vi "Process Messages.vi"(8 "error in (no error)":errorcluster, 11 "Effect in":refnum<class "Effect.lvclass">) -> (0 "error out":errorcluster, 3 "Effect out":refnum<class "Effect.lvclass">)   [LabVIEW 2018, in "Effect.lvclass"]
uses:
  Effect.lvclass
  Effect.lvclass/Effect.ctl
  20a259b6-a1a0-4479-baf0-259017fe30d7.vi
  bbb3d459-c080-460f-b42f-ee43debab906.vi
  Libraries/Messaging/Messaging.lvlib
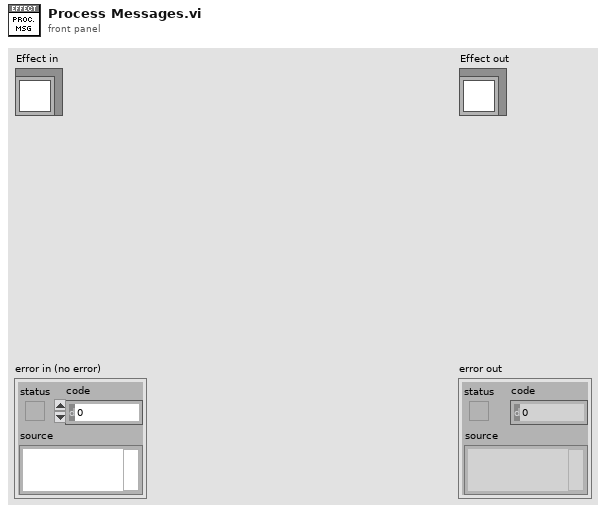
[diagram p1: front panel]
types:
  T1 = typedef "Messaging.lvlib/Message Cluster.ctl" = cluster{"Event":string, "Source":string, "Target":string, "Data":variant}
  T2 = typedef "Audio Processing.lvlib/Value Properties.ctl" = cluster{"Lower":dbl, "Upper":dbl}
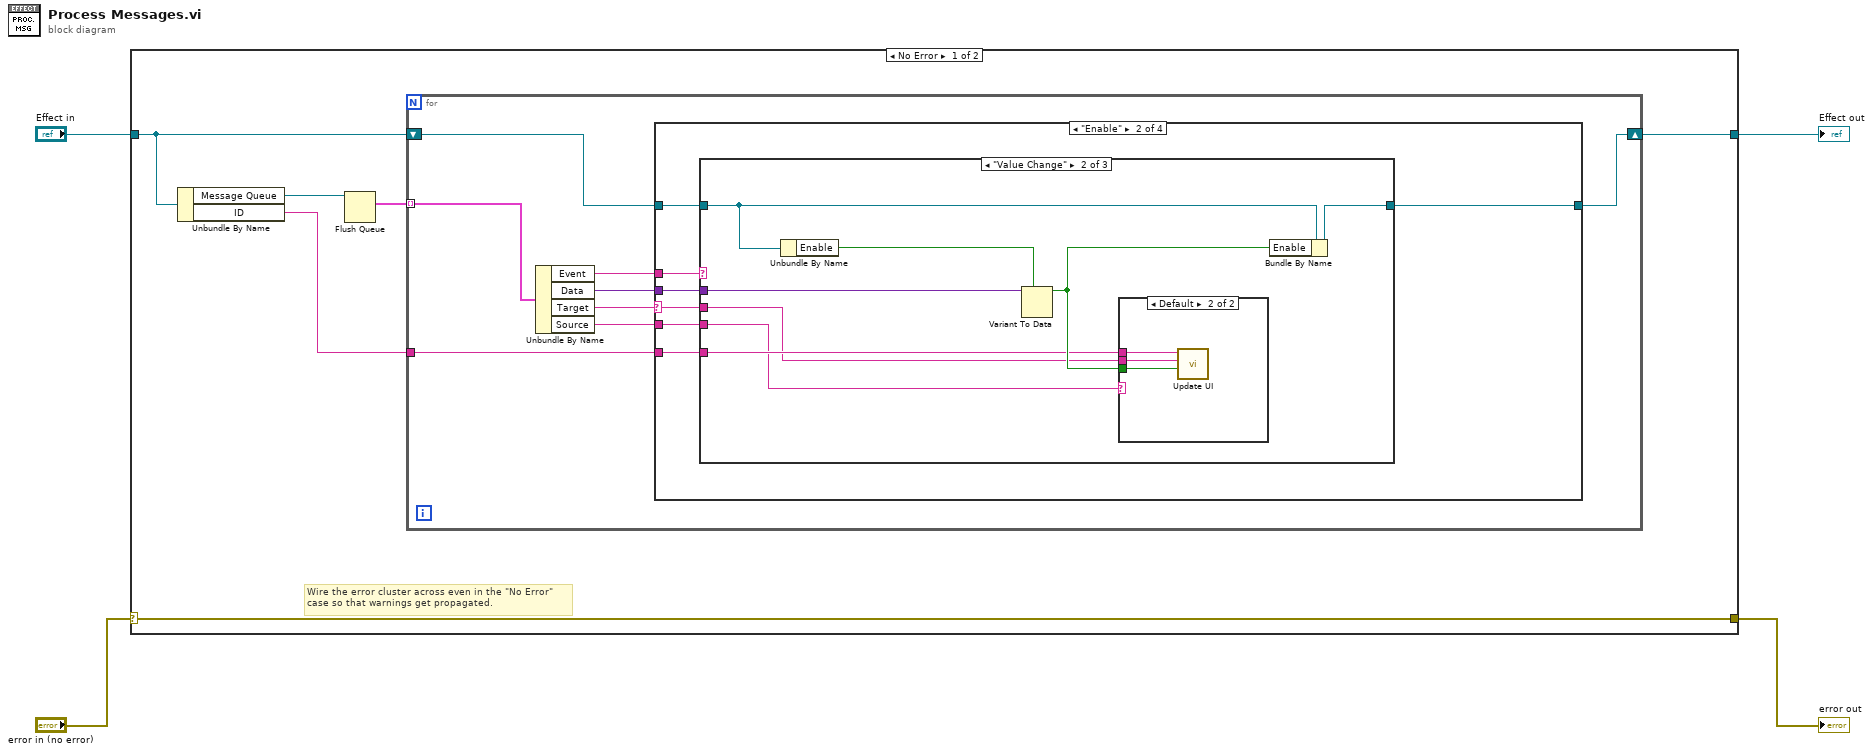
[diagram p0: block diagram]
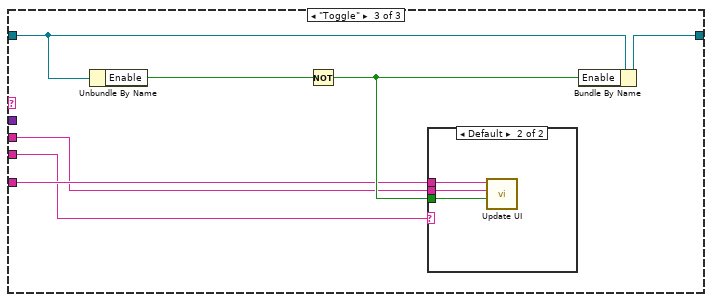
[diagram p5: hidden frame]
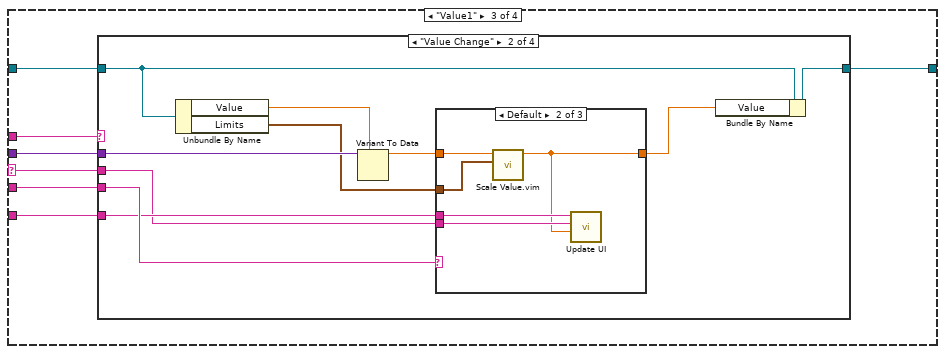
[diagram p7: hidden frame]
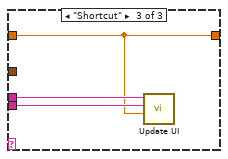
[diagram p10: hidden frame]
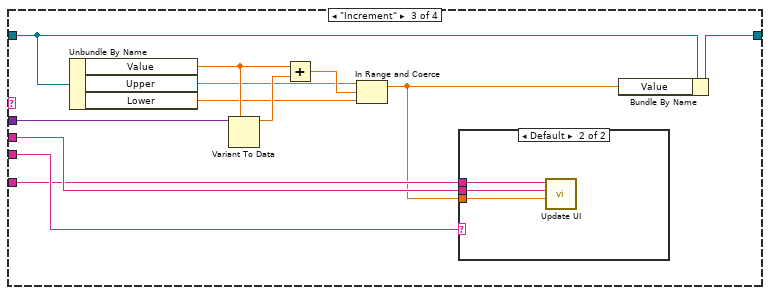
[diagram p11: hidden frame]
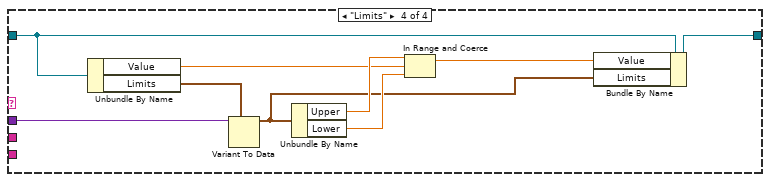
[diagram p13: hidden frame]
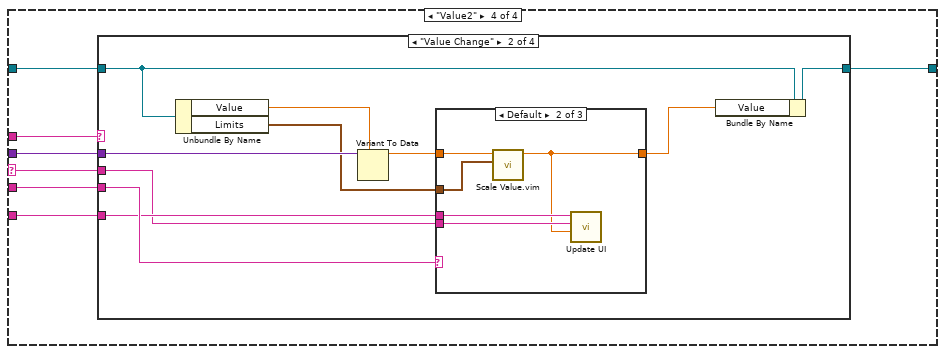
[diagram p14: hidden frame]
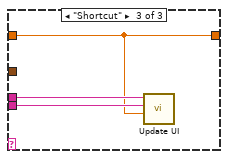
[diagram p17: hidden frame]
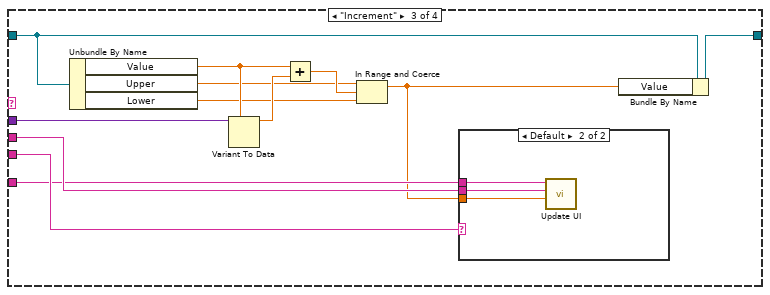
[diagram p18: hidden frame]
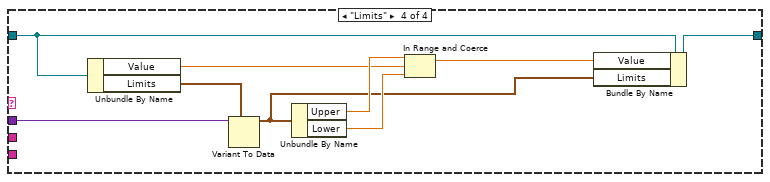
[diagram p20: hidden frame]
diagram:
  n1 = case shown="No Error" "error in (no error)" {
    selector: "error in (no error)" -> [w10 w152]
    tunnel: [w10 w152] -> w1
    tunnel: [w8 w151] -> w3
    tunnel: "Effect in" -> [w9 w151]
    frame No Error {
      # "Wire the error cluster across even in the \"No Error\"\ncase so that warnings get propagated."
      n2 = Unbundle By Name(w9) -> ("Message Queue"=w7:refnum<queue>, "ID"=w5:string)
      n3 = Flush Queue(queue=w7) -> (remaining elements=w6:T1[])  [unwired: 1 in, 2 out]
      n4 = for {
        shift-right: [w15] -> w8
        shift-left: w9 -> [w16]
        tunnel: w6 -> [w18] mode=indexing
        tunnel: w5 -> [w11]
        n5 = Unbundle By Name(w18) -> ("Event"=w14:string, "Data"=w13:variant, "Target"=w17:string, "Source"=w12:string)
        n6 = case shown="\"Enable\"" w17 {
          selector: w17 -> [_ w21 w51 w102]
          tunnel: w16 -> [w19 w25 w55 w105]
          tunnel: [w19 w23 w54 w104] -> w15
          tunnel: w14 -> [_ w26 w53 w106]
          tunnel: w13 -> [_ w24 w52 w103]
          tunnel: w12 -> [_ w22 w49 w101]
          tunnel: w11 -> [_ w20 w50 w100]
          frame Default {
          }
          frame "Enable" {
            n7 = case shown="\"Value Change\"" w26 {
              tunnel: w25 -> [w27 w33 w45]
              tunnel: w24 -> [_ w35 _]
              tunnel: [w27 w32 w44] -> w23
              tunnel: w22 -> [_ w28 w39]
              tunnel: w21 -> [_ w29 w40]
              tunnel: w20 -> [_ w30 w41]
              frame Default {
              }
              frame "Value Change" {
                n8 = Unbundle By Name(w33) -> ("Enable"=w34:bool)
                n9 = Variant To Data(type=w34, Variant=w35) -> (data=w31:bool)  [unwired: 1 in, 1 out]
                n10 = case shown="Default" w28 {
                  tunnel: w30 -> [_ w38]
                  tunnel: w29 -> [_ w37]
                  tunnel: w31 -> [_ w36]
                  frame "UI" {
                  }
                  frame Default {
                    n11 = call "Update UI.vi"("Data"=w36, "Target"=w37, "ID"=w38) -> ()  [unwired: 8 in, 1 out]
                  }
                }
                n12 = Bundle By Name(cluster=w33, "Enable"=w31) -> (w32:refnum<class "Effect.lvclass">)
              }
              frame "Toggle" {
                n13 = Unbundle By Name(w45) -> ("Enable"=w43:bool)
                n14 = Not(x=w43) -> (.not. x?=w42:bool)
                n15 = case shown="Default" w39 {
                  tunnel: w41 -> [_ w48]
                  tunnel: w40 -> [_ w47]
                  tunnel: w42 -> [_ w46]
                  frame "UI" {
                  }
                  frame Default {
                    n16 = call "Update UI.vi"("Data"=w46, "Target"=w47, "ID"=w48) -> ()  [unwired: 8 in, 1 out]
                  }
                }
                n17 = Bundle By Name(cluster=w45, "Enable"=w42) -> (w44:refnum<class "Effect.lvclass">)
              }
            }
          }
          frame "Value1" {
            n18 = case shown="\"Value Change\"" w53 {
              tunnel: [w56 w63 w85 w97] -> w54
              tunnel: w55 -> [w56 w64 w86 w98]
              tunnel: w52 -> [_ w65 w87 w99]
              tunnel: w49 -> [_ w61 w84 _]
              tunnel: w51 -> [_ w59 w83 _]
              tunnel: w50 -> [_ w60 w82 _]
              frame Default {
              }
              frame "Value Change" {
                n19 = Unbundle By Name(w64) -> ("Value"=w66:dbl, "Limits"=w57:T2)
                n20 = Variant To Data(type=w66, Variant=w65) -> (data=w62:dbl)  [unwired: 1 in, 1 out]
                n21 = case shown="Default" w61 {
                  tunnel: w62 -> [w67 w70 w73]
                  tunnel: w59 -> [_ w72 w75]
                  tunnel: w60 -> [_ w71 w74]
                  tunnel: [w67 w68 w73] -> w58
                  tunnel: w57 -> [_ w69 _]
                  frame "UI" {
                  }
                  frame Default {
                    n22 = call "Scale Value.vim"("Limits"=w69, "Value"=w70) -> ("Scaled Value"=w68:dbl)  [unwired: 9 in]
                    n23 = call "Update UI.vi"("Data"=w68, "Target"=w72, "ID"=w71) -> ()  [unwired: 8 in, 1 out]
                  }
                  frame "Shortcut" {
                    n24 = call "Update UI.vi"("Data"=w73, "Target"=w75, "ID"=w74) -> ()  [unwired: 8 in, 1 out]
                  }
                }
                n25 = Bundle By Name(cluster=w64, "Value"=w58) -> (w63:refnum<class "Effect.lvclass">)
              }
              frame "Increment" {
                n26 = Unbundle By Name(w86) -> ("Value"=w81:dbl, "Upper"=w78:dbl, "Lower"=w77:dbl)
                n27 = Variant To Data(type=w81, Variant=w87) -> (data=w80:dbl)  [unwired: 1 in, 1 out]
                n28 = Add(x=w81, y=w80) -> (x+y=w79:dbl)
                n29 = In Range and Coerce(upper limit=w78, x=w79, lower limit=w77) -> (coerced(x)=w76:dbl)  [unwired: 1 out]
                n30 = case shown="Default" w84 {
                  tunnel: w76 -> [_ w90]
                  tunnel: w83 -> [_ w89]
                  tunnel: w82 -> [_ w88]
                  frame "UI" {
                  }
                  frame Default {
                    n31 = call "Update UI.vi"("Data"=w90, "Target"=w89, "ID"=w88) -> ()  [unwired: 8 in, 1 out]
                  }
                }
                n32 = Bundle By Name(cluster=w86, "Value"=w76) -> (w85:refnum<class "Effect.lvclass">)
              }
              frame "Limits" {
                n33 = Unbundle By Name(w98) -> ("Value"=w93:dbl, "Limits"=w91:T2)
                n34 = Variant To Data(type=w91, Variant=w99) -> (data=w92:T2)  [unwired: 1 in, 1 out]
                n35 = Unbundle By Name(w92) -> ("Upper"=w95:dbl, "Lower"=w94:dbl)
                n36 = In Range and Coerce(upper limit=w95, x=w93, lower limit=w94) -> (coerced(x)=w96:dbl)  [unwired: 1 out]
                n37 = Bundle By Name(cluster=w98, "Value"=w96, "Limits"=w92) -> (w97:refnum<class "Effect.lvclass">)
              }
            }
          }
          frame "Value2" {
            n38 = case shown="\"Value Change\"" w106 {
              tunnel: [w107 w114 w136 w148] -> w104
              tunnel: w105 -> [w107 w115 w137 w149]
              tunnel: w103 -> [_ w116 w138 w150]
              tunnel: w101 -> [_ w112 w135 _]
              tunnel: w102 -> [_ w110 w134 _]
              tunnel: w100 -> [_ w111 w133 _]
              frame Default {
              }
              frame "Value Change" {
                n39 = Unbundle By Name(w115) -> ("Value"=w117:dbl, "Limits"=w108:T2)
                n40 = Variant To Data(type=w117, Variant=w116) -> (data=w113:dbl)  [unwired: 1 in, 1 out]
                n41 = case shown="Default" w112 {
                  tunnel: w113 -> [w118 w121 w124]
                  tunnel: w110 -> [_ w123 w126]
                  tunnel: w111 -> [_ w122 w125]
                  tunnel: [w118 w119 w124] -> w109
                  tunnel: w108 -> [_ w120 _]
                  frame "UI" {
                  }
                  frame Default {
                    n42 = call "Scale Value.vim"("Limits"=w120, "Value"=w121) -> ("Scaled Value"=w119:dbl)  [unwired: 9 in]
                    n43 = call "Update UI.vi"("Data"=w119, "Target"=w123, "ID"=w122) -> ()  [unwired: 8 in, 1 out]
                  }
                  frame "Shortcut" {
                    n44 = call "Update UI.vi"("Data"=w124, "Target"=w126, "ID"=w125) -> ()  [unwired: 8 in, 1 out]
                  }
                }
                n45 = Bundle By Name(cluster=w115, "Value"=w109) -> (w114:refnum<class "Effect.lvclass">)
              }
              frame "Increment" {
                n46 = Unbundle By Name(w137) -> ("Value"=w132:dbl, "Upper"=w129:dbl, "Lower"=w128:dbl)
                n47 = Variant To Data(type=w132, Variant=w138) -> (data=w131:dbl)  [unwired: 1 in, 1 out]
                n48 = Add(x=w132, y=w131) -> (x+y=w130:dbl)
                n49 = In Range and Coerce(upper limit=w129, x=w130, lower limit=w128) -> (coerced(x)=w127:dbl)  [unwired: 1 out]
                n50 = case shown="Default" w135 {
                  tunnel: w127 -> [_ w141]
                  tunnel: w134 -> [_ w140]
                  tunnel: w133 -> [_ w139]
                  frame "UI" {
                  }
                  frame Default {
                    n51 = call "Update UI.vi"("Data"=w141, "Target"=w140, "ID"=w139) -> ()  [unwired: 8 in, 1 out]
                  }
                }
                n52 = Bundle By Name(cluster=w137, "Value"=w127) -> (w136:refnum<class "Effect.lvclass">)
              }
              frame "Limits" {
                n53 = Unbundle By Name(w149) -> ("Value"=w144:dbl, "Limits"=w142:T2)
                n54 = Variant To Data(type=w142, Variant=w150) -> (data=w143:T2)  [unwired: 1 in, 1 out]
                n55 = Unbundle By Name(w143) -> ("Upper"=w146:dbl, "Lower"=w145:dbl)
                n56 = In Range and Coerce(upper limit=w146, x=w144, lower limit=w145) -> (coerced(x)=w147:dbl)  [unwired: 1 out]
                n57 = Bundle By Name(cluster=w149, "Value"=w147, "Limits"=w143) -> (w148:refnum<class "Effect.lvclass">)
              }
            }
          }
        }
      }
    }
    frame Error {
    }
  }
  "error out" <- w1
  "Effect out" <- w3
